vi "Page_Source_Supports_Configurable_VI.vi"(8 "error in (no error)":errorcluster, 11 "AB_DLL in":refnum<class "AB_DLL.lvclass">) -> (0 "error out":errorcluster, 2 "supports configurable VI":bool, 3 "AB_DLL out":refnum<class "AB_DLL.lvclass">)   [LabVIEW 2020, in "AB_DLL.lvclass"]
uses:
  <vilib>/AppBuilder/AB_Classes/DLL/AB_DLL.lvclass
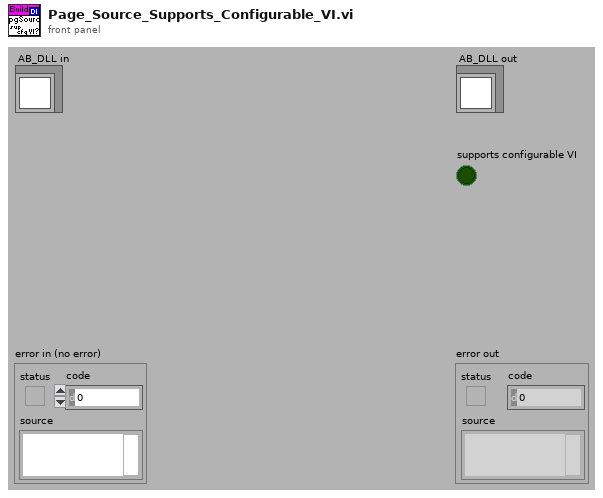
[diagram p1: front panel]
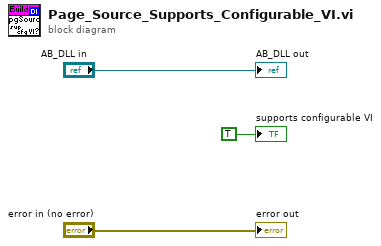
[diagram p0: block diagram]
diagram:
  "error out" <- "error in (no error)"
  "AB_DLL out" <- "AB_DLL in"
  "supports configurable VI" <- TRUE ("supports configurable VI")
